vi "Install Dependencies.vi"(0 "NIPKG_LV in":refnum<class "NIPKG_LV.lvclass">) -> (4 "NIPKG_LV out":refnum<class "NIPKG_LV.lvclass">)   [LabVIEW 2017, in "CL_G3_VIComponentBuilder.lvlib" / "NIPKG_LV.lvclass"]
doc: "Installs the dependencies required by this export at build time."
uses:
  NIPKG_LV.lvclass
  C:/Tool Chain Support/Software Module Builder/Source/Exports/NI Build Specification_LV/NI Build Specification_LV.lvclass
  C:/Tool Chain Support/Software Module Builder/Source/Exports/Exports/Export.lvclass
  NI Build Specification_LV/NI Build Specification_LV.lvclass/NI Build Specification_LV.ctl
  Exports/Export.lvclass/Export.ctl
  <userlib>/_Cirrus Logic/NI Package Manager API/Source/Version Comparison Operator.ctl
  Exports/Accessors/Write Export Operation Errors.vi
  NI Build Specification_LV/Accessors/Read Project Reference.vi
  NI Build Specification_LV/Accessors/Read Build Spec Ref.vi
  Exports/Accessors/Read Export Operation Errors.vi
  <userlib>/_Cirrus Logic/NI Package Manager API/Source/TCS_NIPKG_API.lvlib
  <userlib>/_Cirrus Logic/NI Package Manager BldSpec Utils/Source/NIPKG BuildSpec API.lvlib
  <vilib>/National Instruments/NIPM API (Beta)/NIPM_API.lvlib
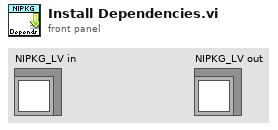
[diagram p1: front panel]
types:
  T1 = typedef "TCS_NIPKG_API.lvlib/Version Comparison Operator.ctl" = enum16{">", ">=", "=", "!=", "<=", "<"}
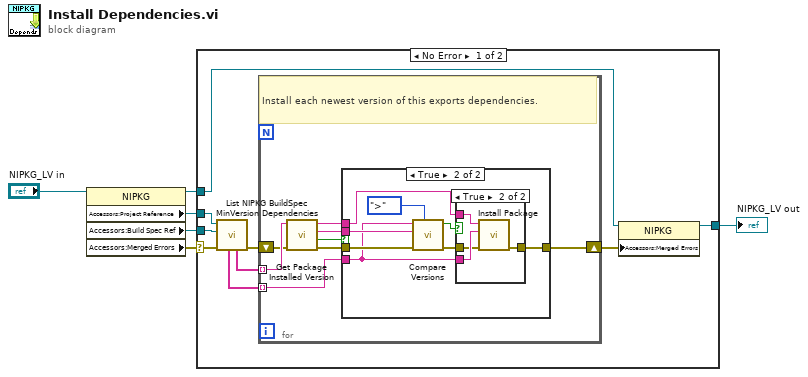
[diagram p0: block diagram]
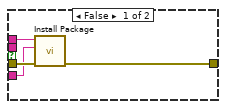
[diagram p2: hidden frame]
diagram:
  n1 = property class="NIPKG"(reference="NIPKG_LV in") -> (reference out=w5:refnum<class "NIPKG_LV.lvclass">, "Accessors:Project Reference"=w3:refnum<vi>, "Accessors:Build Spec Ref"=w2:refnum<vi>, "Accessors:Merged Errors"=w1:errorcluster)  [unwired: 1 in, 1 out]
  n2 = case shown="No Error" w1 {
    selector: w1 -> [w7 _]
    tunnel: w5 -> [w15 w41]
    tunnel: [w14 w41] -> w4
    tunnel: w3 -> [w9 _]
    tunnel: w2 -> [w8 _]
    frame No Error {
      n3 = call <userlib>:"List NIPKG BuildSpec MinVersion Dependencies.vi"("error in (no error)"=w7, "package buildspec ref in"=w8, "project ref in"=w9) -> ("error out"=w10:errorcluster, "dependency package names"=w12:string[], "dependency package min versions"=w11:string[])  [unwired: 4 in, 2 out]
      n4 = for {
        tunnel: w12 -> [w22] mode=indexing
        tunnel: w11 -> [w17] mode=indexing
        shift-right: [w23] -> w13
        shift-left: w10 -> [w20]
        # "Install each newest version of this exports dependencies."
        n5 = call <vilib>:"Get Package Installed Version.vi"("error in"=w20, "package name"=w22) -> ("error out"=w19:errorcluster, "installed?"=w16:bool, "installed version"=w21:string, "package name out"=w18:string)  [unwired: 6 in]
        n6 = case shown="True" w16 {
          tunnel: [w26 w35] -> w23
          tunnel: w21 -> [_ w33]
          tunnel: w19 -> [w27 w32]
          tunnel: w17 -> [w24 w30]
          tunnel: w18 -> [w25 w28]
          frame False {
            n7 = call <vilib>:"Install Package.vi"("error in"=w27, "version"=w24, "package name"=w25) -> ("error out"=w26:errorcluster)  [unwired: 8 in]
          }
          frame True {
            n8 = call <userlib>:"Compare Versions.vi"("operator"=Version_Comparison_Operator.">", "error in"=w32, "version y"=w33, "version x"=w30) -> ("error out"=w31:errorcluster, "Satisfied?"=w29:bool)  [unwired: 6 in]
            n9 = case shown="True" w29 {
              tunnel: w28 -> [_ w39]
              tunnel: [w36 w37] -> w35
              tunnel: w31 -> [w36 w38]
              tunnel: w30 -> [_ w40]
              frame False {
              }
              frame True {
                n10 = call <vilib>:"Install Package.vi"("error in"=w38, "version"=w40, "package name"=w39) -> ("error out"=w37:errorcluster)  [unwired: 6 in, 2 out]
              }
            }
          }
        }
      }
      n11 = property class="NIPKG"(reference=w15, "Accessors:Merged Errors"=w13) -> (reference out=w14:refnum<class "NIPKG_LV.lvclass">)  [unwired: 1 in, 1 out]
    }
    frame Error {
    }
  }
  "NIPKG_LV out" <- w4
